vi "DI Post Step.vi"(8 "error in (no error)":errorcluster, 9 "DI In":T1, 10 "Socket No":u16=1, 11 "NI Digital Input in":refnum<class "NI Digital Input.lvclass">) -> (0 "error out":errorcluster, 1 "AnalogRead":bool[](array[boolean]), 2 "Report Text":string, 3 "NI Digital Input out":refnum<class "NI Digital Input.lvclass">, 4 "PhysicalChannel":string[](array[string]))   [LabVIEW 2023, in "HardwareAbstractionLayer_LVOOP.lvlib" / "NI Digital Input.lvclass"]
uses:
  NI Digital Input.lvclass
  DI_class/DI DAQ/Control/DI Step Control.ctl
  NI Digital Input.lvclass/NI Digital Input.ctl
  Database/Database.lvclass
  <resource>/objmgr/daqmx.rc
  DI_class/DI.lvclass
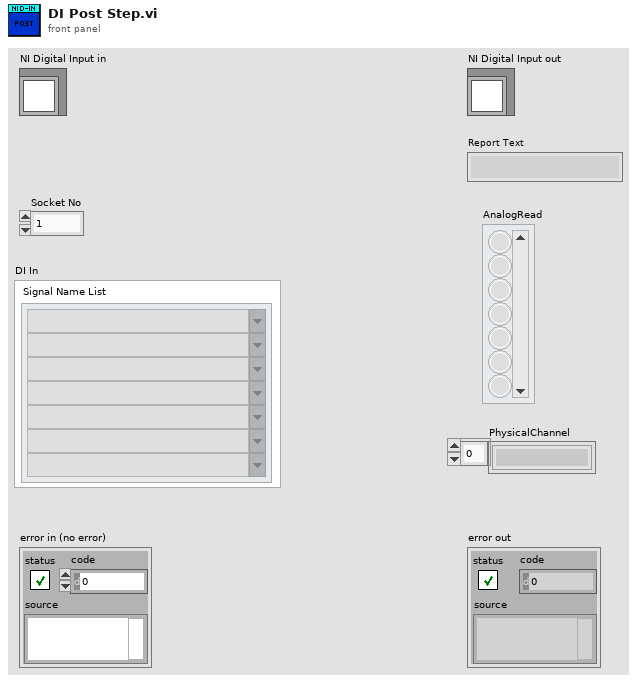
[diagram p1: front panel]
types:
  T1 = typedef "HardwareAbstractionLayer_LVOOP.lvlib/DI.lvclass/DI Step Control.ctl" = cluster{"Signal Name List":string[]}
  T2 = cluster{"table":string, "condition":string, "columns":string[]}
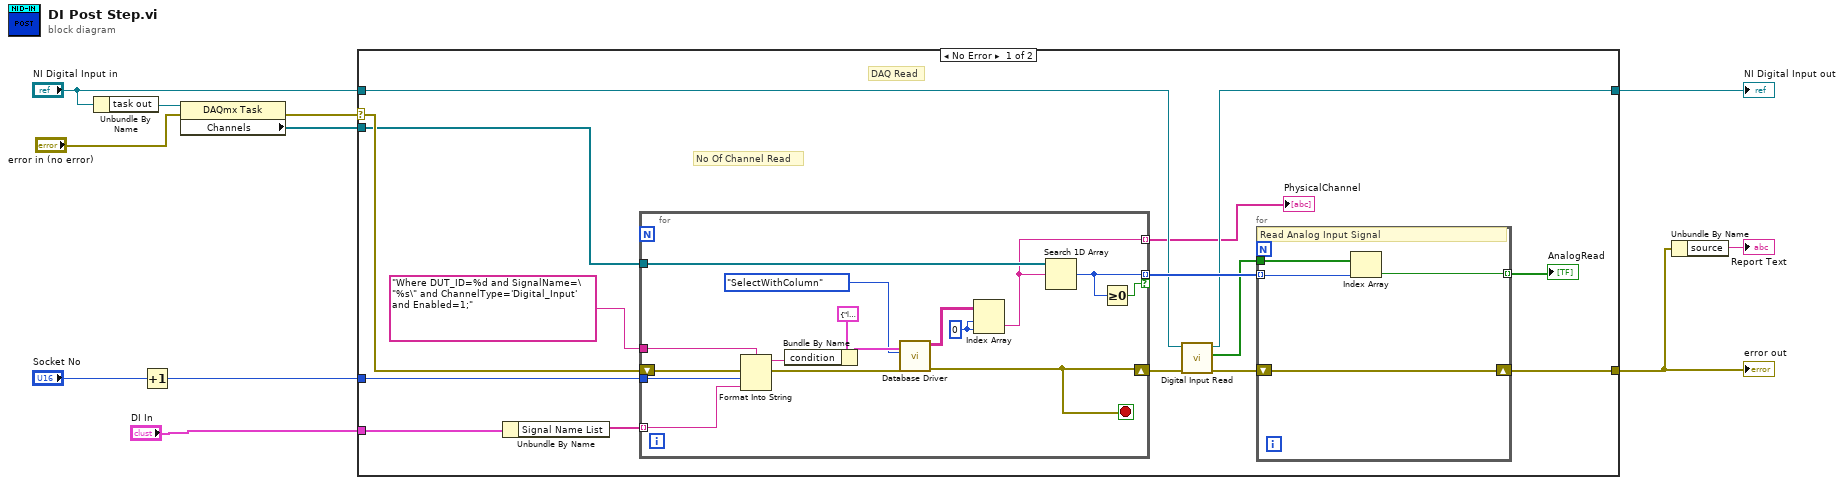
[diagram p0: block diagram]
diagram:
  n1 = Unbundle By Name("NI Digital Input in") -> ("task out"=w11:refnum<k21>)
  n2 = Increment(x="Socket No") -> (x+1=w4:u16)
  n3 = property class="DAQmx Task"(reference=w11, error in="error in (no error)") -> (error out=w2:errorcluster, "Channels"=w9:refnum<k21>[])  [unwired: 1 out]
  n4 = case shown="No Error" w2 {
    selector: w2 -> [w20 w47]
    tunnel: [w26 w47] -> w6
    tunnel: "DI In" -> [w25 _]
    tunnel: w4 -> [w21 _]
    tunnel: w9 -> [w19 _]
    tunnel: "NI Digital Input in" -> [w18 w48]
    tunnel: [w14 w48] -> w7
    frame No Error {
      # "No Of Channel Read"
      # "DAQ Read"
      n5 = Unbundle By Name(w25) -> ("Signal Name List"=w24:string[])
      n6 = for {
        tunnel: w24 -> [w40] mode=indexing
        tunnel: "Where DUT_ID=%d and SignalName=\"%s\" and ChannelType='Digital_Input' and Enabled=1;" -> [w42]
        tunnel: w21 -> [w41]
        shift-right: [w30] -> w17
        shift-left: w20 -> [w36]
        tunnel: [w32] -> w22 mode=indexing if=w31
        tunnel: w19 -> [w28]
        tunnel: [w27] -> w12 mode=indexing
        stop <- w30 stop-if-true
        w33 = 0 ("disabled index (col)")
        n7 = Format Into String(format string=w42, error in=w36, w41, w40) -> (resulting string=w38:string, error out=w35:errorcluster)  [unwired: 1 in]
        n8 = Bundle By Name(cluster=T2 {"table"="ltt.daq_configuration", "condition"="Where ChannelType='Analog_Input' and Enabled=1", "columns"=["PhysicalChannel"]} ("SQLTableData"), "condition"=w38) -> (w37:T2)
        n9 = call "Database Driver.vi"("SQLTableData"=w37, "error in"=w35, "Select"=enum16{"SelectWithQuery", "SelectWithColumn"}."SelectWithColumn") -> ("error out"=w30:errorcluster, "data"=w34:string[][])  [unwired: 5 in, 2 out]
        n10 = Index Array(array=w34, index (row)=w33, index (col)=w33) -> (element=w27:string)
        n11 = Search 1D Array(1D array=w28, element=w27) -> (index of element=w32:i32)  [unwired: 1 in]
        n12 = Greater Or Equal To 0?(x=w32) -> (x >= 0?=w31:bool)
      }
      "PhysicalChannel" <- w12
      n13 = call-dynamic "Digital Input Read.vi"("error in (no error)"=w17, "NI Digital Input in"=w18) -> ("error out"=w16:errorcluster, "data"=w15:bool[], "NI Digital Input out"=w14:refnum<class "NI Digital Input.lvclass">)  [unwired: 7 in]
      n14 = for {
        shift-right: [w46] -> w26
        shift-left: w16 -> [w46]
        tunnel: w15 -> [w45]
        tunnel: w22 -> [w44] mode=indexing
        tunnel: [w43] -> w13 mode=indexing
        # "Read Analog Input Signal"
        n15 = Index Array(array=w45, index=w44) -> (element=w43:bool)
      }
      "AnalogRead" <- w13
    }
    frame Error {
    }
  }
  "error out" <- w6
  "NI Digital Input out" <- w7
  n16 = Unbundle By Name(w6) -> ("source"=→"Report Text":string)
